vi "Set DateTimeOrginal.vi"() -> ()   [LabVIEW 2023]
panel:
  out "x+y":timestamp
  out "x-y":dbl
  in  "Time Stamp 2":timestamp
  in  "Time Stamp":timestamp
  out "error out":errorcluster
  out "standard error":string
  in  "Path":path
  out "output 1":timestamp
  out "after substring":string
  out "standard output":string
  # "Date/Time Original              : 2011:03:08 19:53:18"
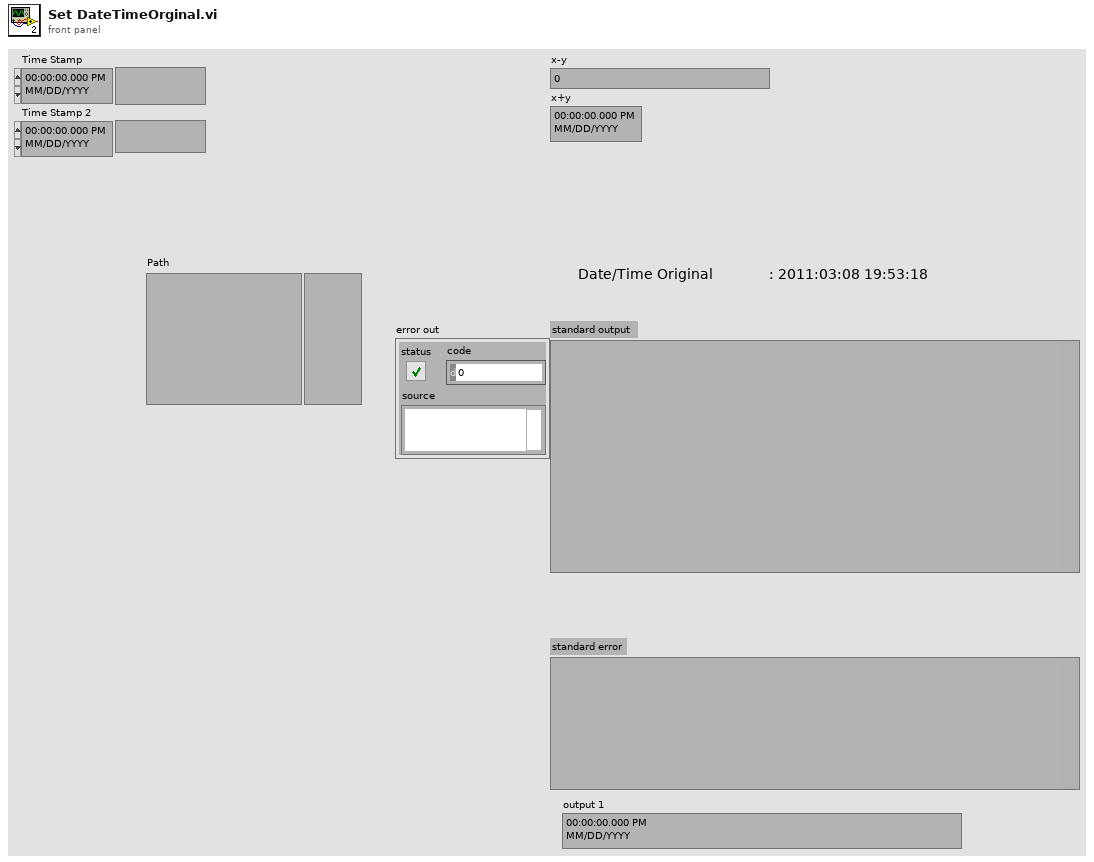
[diagram p1: front panel]
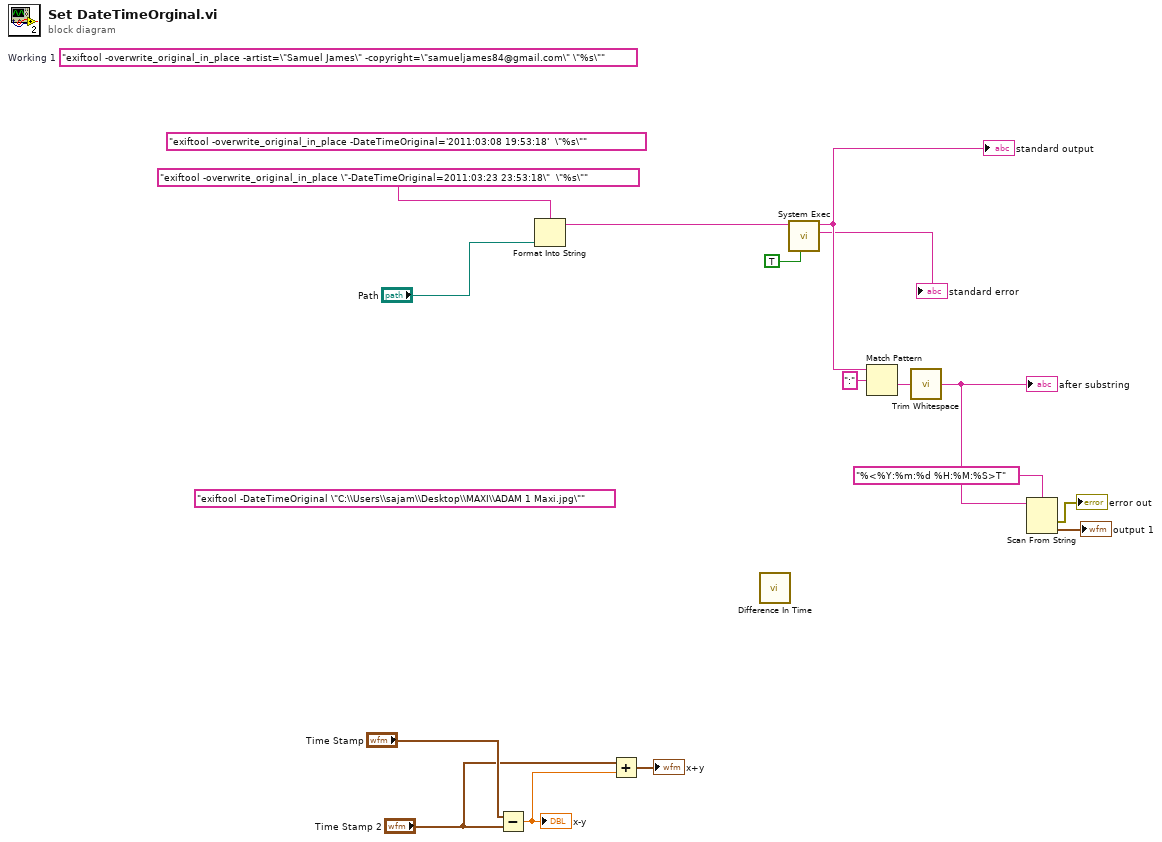
[diagram p0: block diagram]
diagram:
  (unwired) "exiftool -overwrite_original_in_place -artist=\"Samuel James\" -copyright=\"samueljames84@gmail.com\" \"%s\""  # Working 1
  (unwired) "exiftool -overwrite_original_in_place -DateTimeOriginal='2011:03:08 19:53:18'  \"%s\"" ("command line")
  (unwired) "exiftool -DateTimeOriginal \"C:\\Users\\sajam\\Desktop\\MAXI\\ADAM 1 Maxi.jpg\"" ("standard input")
  n1 = Subtract(x="Time Stamp", y="Time Stamp 2") -> (x-y=w4:dbl)
  "x-y" <- w4
  n2 = Format Into String(format string="exiftool -overwrite_original_in_place \"-DateTimeOriginal=2011:03:23 23:53:18\"  \"%s\"" ("command line"), "Path") -> (resulting string=w7:string)  [unwired: 2 in, 1 out]
  n3 = Add(x="Time Stamp 2", y=w4) -> (x+y=→"x+y":timestamp)
  n4 = call "Difference In Time.vi"() -> ()  [unwired: 12 in]
  n5 = call <vilib>:"System Exec.vi"("run minimized? (F)"=TRUE, "command line"=w7) -> ("standard error"=→"standard error":string, "standard output"=w15:string)  [unwired: 6 in, 2 out]
  "standard output" <- w15
  n6 = Match Pattern(string=w15, regular expression=":") -> (after substring=w13:string)  [unwired: 1 in, 3 out]
  n7 = call <vilib>:"Trim Whitespace.vi"("string"=w13) -> ("trimmed string"=w10:string)  [unwired: 1 in]
  "after substring" <- w10
  n8 = Scan From String(format string="%<%Y:%m:%d %H:%M:%S>T", input string=w10) -> (error out=→"error out":errorcluster, output 1=→"output 1":timestamp)  [unwired: 3 in, 2 out]
